vi "GT Compare Status.vi"(8 "error in (no error)":errorcluster caption="错误输入（无错误）", 10 "pStatus":i16, 11 "cardNum":i16) -> (0 "error out":errorcluster caption="错误输出", 1 "pCount out":i32[](array[numeric]), 2 "pStatus out":i16, 3 "function return":i16)   [LabVIEW 2020, in "gts.lvlib"]
doc: "GT_API GT_CompareStatus(short cardNum,short *pStatus,long *pCount);"
uses:
  gts.lvlib
  dll/32bit/multi_card/gts.dll
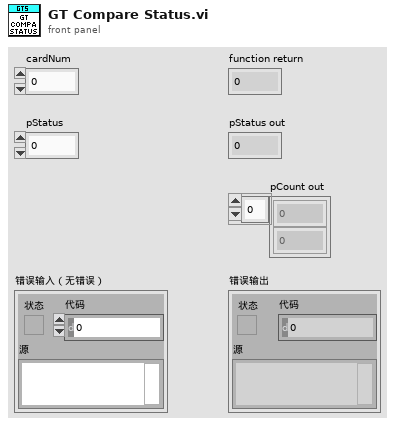
[diagram p1: front panel]
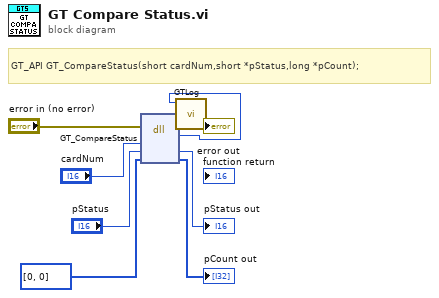
[diagram p0: block diagram]
diagram:
  # "GT_API GT_CompareStatus(short cardNum,short *pStatus,long *pCount);"
  n1 = dll-call lib="C:/1228/dll/32bit/multi_card/gts.dll" fn="GT_CompareStatus"(error in="error in (no error)", "cardNum"="cardNum", "pStatus"="pStatus", "pCount"=i32[] [0, 0]) -> (error out=w3:errorcluster, "返回类型"=w1:i16, "pStatus"=→"pStatus out":i16, "pCount"=→"pCount out":i32[])  [unwired: 3 in, 1 out]
  n2 = call "GTLog.vi"("error in (no error)"=w3, "Numeric"=w1) -> ("error out"=→"error out":errorcluster)  [unwired: 9 in]
